vi "Edgertronic-:get_caminfo copy.vi"(5 "Setup":T2={"URL"="130.64.16.195", "remote port"=80, "mode (standard)"=enum."Standard"}) -> (0 "error out":errorcluster, 1 "Cam Info":T1={"Build Date"="20140911165611", "Software Build Date"="20140911165611", "FPGA Initialized"="20140911165611", "Hardware Revision"="20140911165611", "Model Number"="20140911165611", "Home Dir"="20140911165611", "IR Filter"="20140911165611", "Mac Address"="20140911165611", "Serial Console Enabled"="20140911165611", "Serial number"="20140911165611", "FPGA Version"="20140911165611", "Hardware Configuration"="20140911165611", "Connection Information:"=""}, 2 "data out":string="HTTP/1.0 200 OK\r\nContent-Type: text/html; charset=utf-8\r\nContent-Length: 313\r\nConnection: close\r\nDate: Tue, 16 Jun 2015 13:54:12 GMT\r\nServer: lighttpd/1.4.11 (edgertonic slow motion camera)\r\n\r\n{\"build_date\": \"20150112\", \"sw_build_date\": \"20140911165611\", \"fpga_initialized\": 1, \"hardware_revision\": 6, \"model_number\": 1, \"home_dir\": \"/home/root/ss-web\", \"ir_filter\": 1, \"mac_addr\": \"00:1B:C5:09:61:4D\", \"serial_console_enabled\": false, \"serial_number\": 333, \"fpga_version\": 70, \"hardware_configuration\": 1}")   [LabVIEW 2012]
doc: "This VI returns all the static camera information."
panel:
  in  "GET Cmd":string="/get_caminfo"
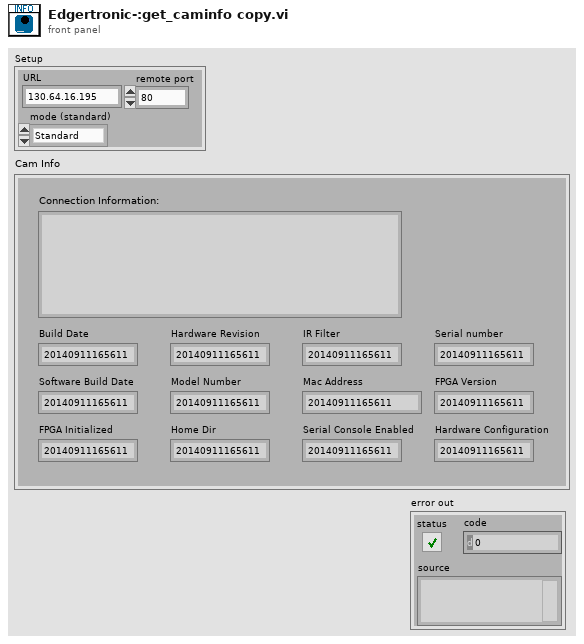
[diagram p1: front panel]
types:
  T1 = cluster{"Build Date":string, "Software Build Date":string, "FPGA Initialized":string, "Hardware Revision":string, "Model Number":string, "Home Dir":string, "IR Filter":string, "Mac Address":string, "Serial Console Enabled":string, "Serial number":string, "FPGA Version":string, "Hardware Configuration":string, "Connection Information:":string}
  T2 = cluster{"URL":string, "remote port":u16, "mode (standard)":enum16{"Standard", "Buffered", "CRLF", "Immediate"}}
  T3 = cluster{"Parameter":string, "Parameter 2":string, "Parameter 3":string, "Parameter 4":string, "Parameter 5":string, "Parameter 6":string, "Parameter 7":string, "Parameter 8":string, "Parameter 9":string, "Parameter 10":string, "Parameter 11":string, "Parameter 12":string, "Parameter 13":string, "Parameter 14":string, "Parameter 15":string, "Parameter 16":string, "Parameter 17":string, "Parameter 18":string, "Parameter 19":string, "Parameter 20":string, "Parameter 21":string, "Parameter 22":string, "Parameter 23":string, "Parameter 24":string, "Parameter 25":string, "Parameter 26":string, "Parameter 27":string, "Parameter 28":string, "Parameter 29":string, "Parameter 30":string, "Parameter 31":string, "Parameter 32":string, "Parameter 33":string, "Parameter 34":string, "Parameter 35":string, "Parameter 36":string}
  T4 = cluster{"[0]":string, "[1]":string, "[2]":string, "[3]":string, "[4]":string, "[5]":string, "[6]":string, "[7]":string, "[8]":string, "[9]":string, "[10]":string, "[11]":string, "[12]":string, "[13]":string, "[14]":string, "[15]":string, "[16]":string, "[17]":string, "[18]":string, "[19]":string, "[20]":string, "[21]":string, "[22]":string, "[23]":string, "[24]":string, "[25]":string, "[26]":string, "[27]":string, "[28]":string, "[29]":string, "[30]":string, "[31]":string, "[32]":string, "[33]":string, "[34]":string, "[35]":string}
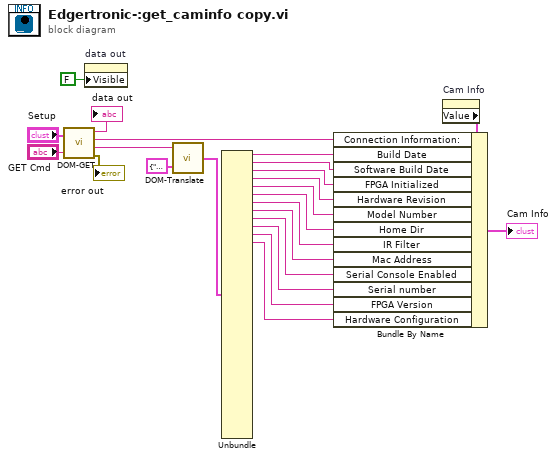
[diagram p0: block diagram]
diagram:
  n1 = call <userlib>:"DOM-GET.vi"("Setup"="Setup", "GET Command"="GET Cmd") -> ("Data Out from Camera"=→"data out":string, "Connection Information"=w16:string, "Value String"=w15:string, "error out"=→"error out":errorcluster)
  n2 = property on="data out" class="Str"("Visible"=FALSE) -> ()  [unwired: 2 in, 2 out]
  n3 = call <userlib>:"DOM-Translate.vi"("Parameter Cluster in"=T3 {"Parameter"="build_date", "Parameter 2"="sw_build_date", "Parameter 3"="fpga_initialized", "Parameter 4"="hardware_revision", "Parameter 5"="model_number", "Parameter 6"="home_dir", "Parameter 7"="ir_filter", "Parameter 8"="mac_addr", "Parameter 9"="serial_console_enabled", "Parameter 10"="serial_number", "Parameter 11"="fpga_version", "Parameter 12"="hardware_configuration", "Parameter 13"=" ", "Parameter 14"=" ", "Parameter 15"=" ", "Parameter 16"=" ", "Parameter 17"=" ", "Parameter 18"=" ", "Parameter 19"=" ", "Parameter 20"=" ", "Parameter 21"=" ", "Parameter 22"=" ", "Parameter 23"=" ", "Parameter 24"=" ", "Parameter 25"=" ", "Parameter 26"=" ", "Parameter 27"=" ", "Parameter 28"=" ", "Parameter 29"=" ", "Parameter 30"=" ", "Parameter 31"=" ", "Parameter 32"=" ", "Parameter 33"=" ", "Parameter 34"=" ", "Parameter 35"=" ", "Parameter 36"=" "}, "Value Data in"=w15) -> ("Value Cluster out"=w13:T4)
  n4 = Unbundle(w13) -> ("[0]"=w12:string, "[1]"=w11:string, "[2]"=w10:string, "[3]"=w9:string, "[4]"=w8:string, "[5]"=w7:string, "[6]"=w6:string, "[7]"=w5:string, "[8]"=w4:string, "[9]"=w3:string, "[10]"=w2:string, "[11]"=w1:string)  [unwired: 24 out]
  n5 = property on="Cam Info" class="Clust (strict)"() -> ("Value"=w17:T1)  [unwired: 2 in, 2 out]
  n6 = Bundle By Name(cluster=w17, "Connection Information:"=w16, "Build Date"=w12, "Software Build Date"=w11, "FPGA Initialized"=w10, "Hardware Revision"=w9, "Model Number"=w8, "Home Dir"=w7, "IR Filter"=w6, "Mac Address"=w5, "Serial Console Enabled"=w4, "Serial number"=w3, "FPGA Version"=w2, "Hardware Configuration"=w1) -> (→"Cam Info":T1)
